vi "Example - Class.vi"() -> ()   [LabVIEW 2020]
uses:
  1d4a776c-2696-3fe4-d0bb-77cddb30cb3f.vi
  3faee846-98d4-3fe1-9c43-23fda36bd13f.vi
  b5272922-ba09-3fe1-f861-5bbbaacdd13f.vi
  EquipmentVariant/Type Enum.ctl
  EquipmentVariant/EquipmentVariant.lvclass
  fdb528fa-7372-3fe0-10ac-5ff425bcdf3f.vi
  49be02a8-6884-3fd8-d48e-5d860b02e23f.vi
  cd560766-33b7-3fed-e07d-7da03414de3f.vi
  d5be5900-83d0-3fd0-7918-a6c719c6ef3f.vi
  70d5f8a8-1432-3fec-90d8-8f9e559dd13f.vi
  6e1ed180-022c-3fcd-f5ed-a54cfad1e83f.vi
  092b700a-44bb-3fe9-485c-b2951c1cd43f.vi
  43438abc-0b96-3fe5-e002-a3a3c6ecc43f.vi
  682f44c6-7f56-3fe3-7cfd-dfadc80bee3f.vi
  2733e0e4-24d6-3fee-700d-63818caedb3f.vi
  915d7a80-1a4e-3fce-50ff-63604885b63f.vi
  Robot/Robot.lvclass
  Pump/Pump.lvclass
  45b58a9c-ccc2-3fe8-f4b2-f6788901e33f.vi
  36c48e48-6b2d-3fef-c04d-7500d28fc73f.vi
  507d9734-094a-3fee-fad7-d41d2ba6e43f.vi
  home/jki/Projects/enumerated-variant-labview-idea/source/EnumeratedVariant/EnumeratedVariant.lvclass
  home/jki/Projects/enumerated-variant-labview-idea/source/EquipmentVariant/EquipmentVariant.lvclass
  75226f00-6cff-3fc0-1085-64b70facdd3f.vi
  1b391bf8-c4d0-3fd5-10eb-bf28fd58bc3f.vi
  dfc18360-e89b-3fe8-f7d0-384086f7e73f.vi
  a19e52fe-f2f8-3fee-80fa-777f1c989c3f.vi
  b0de32f8-392d-3fea-f061-38c88206d93f.vi
  47083128-469b-3fd6-4083-c0c0298ca53f.vi
  f64f6dae-26cd-3fe7-164d-c343c130e33f.vi
  d52d8690-3443-3fb2-48a2-82c20901ea3f.vi
  9c66e4d8-756c-3fe3-f899-0197e0a0e13f.vi
  fbe86e10-61e9-3fd4-3453-d6eec0f7ec3f.vi
  bcedb830-bb68-3fd0-605d-ec66737db43f.vi
  9f07b280-4224-3fc7-a086-75c6439fc93f.vi
  efe137e0-dc7b-3fc0-d86a-56f12716df3f.vi
  5fb9f880-a967-3fa0-c07e-0f50a7d0c93f.vi
  65dfe200-eb14-3fe5-806e-08bf00ddc13f.vi
panel:
  in  "error in":errorcluster
  out "error out":errorcluster
  out "Pump 3":refnum<class "Pump.lvclass">
  out "Robot 4":refnum<class "Robot.lvclass">
  out "Equipment Array":refnum<class "EquipmentVariant.lvclass">[](array[class])
  out "Pump 2":refnum<class "Pump.lvclass">
  out "Robot 3":refnum<class "Robot.lvclass">
  out "Pump":refnum<class "Pump.lvclass">
  out "Robot 2":refnum<class "Robot.lvclass">
  out "Pump":refnum<class "Pump.lvclass">
  out "Robot":refnum<class "Robot.lvclass">
  out "Pump":refnum<class "Pump.lvclass">
  out "Robot":refnum<class "Robot.lvclass">
  out "specific type":refnum<visa-resource-name>="abc"
  out "specific type":refnum<class "Pump.lvclass">
  out "specific type":refnum<class "Robot.lvclass">
  out "Pump":refnum<class "Pump.lvclass">
  out "Robot":refnum<class "Robot.lvclass">
  out "Pump":refnum<class "Pump.lvclass">
  out "Robot":refnum<class "Robot.lvclass">
  out "Equivalent?":bool
  out "Equivalent?":bool
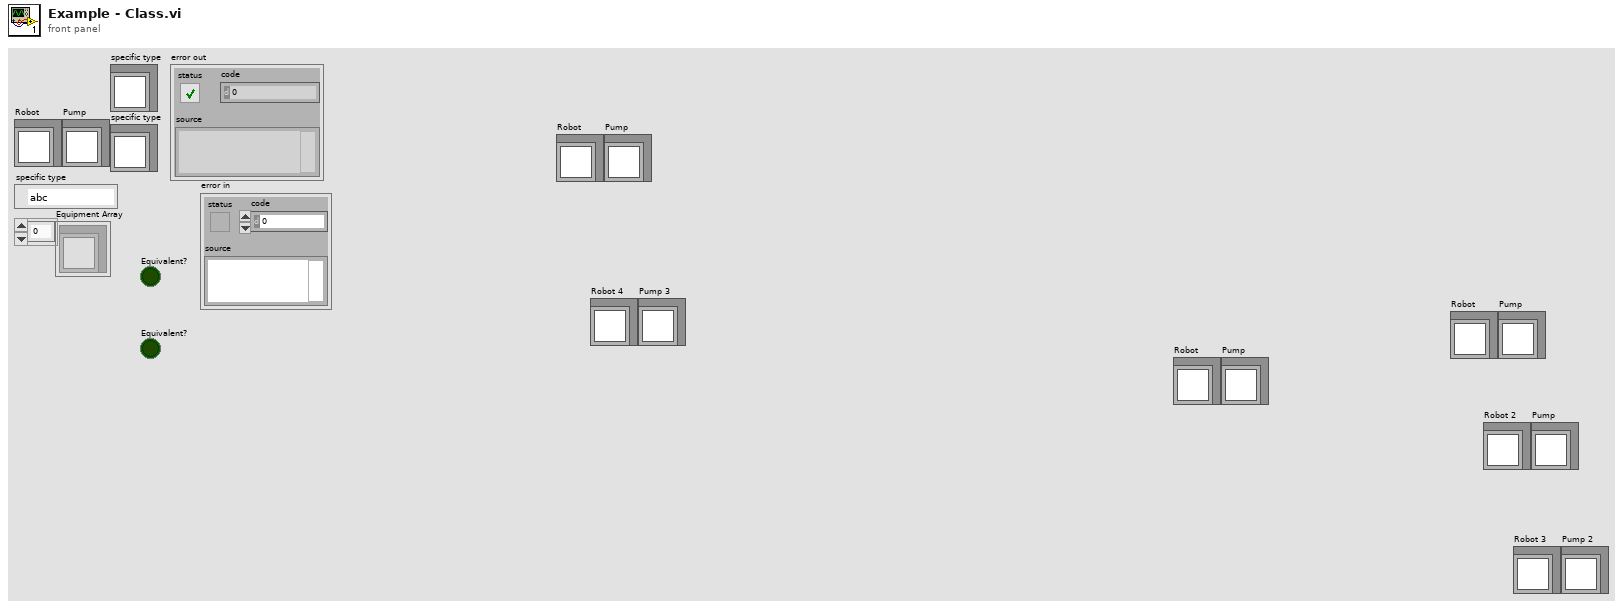
[diagram p1: front panel]
types:
  T1 = typedef "EquipmentVariant.lvclass/Type Enum.ctl" = enum16{"Robot", "Pump", "Instrument"}
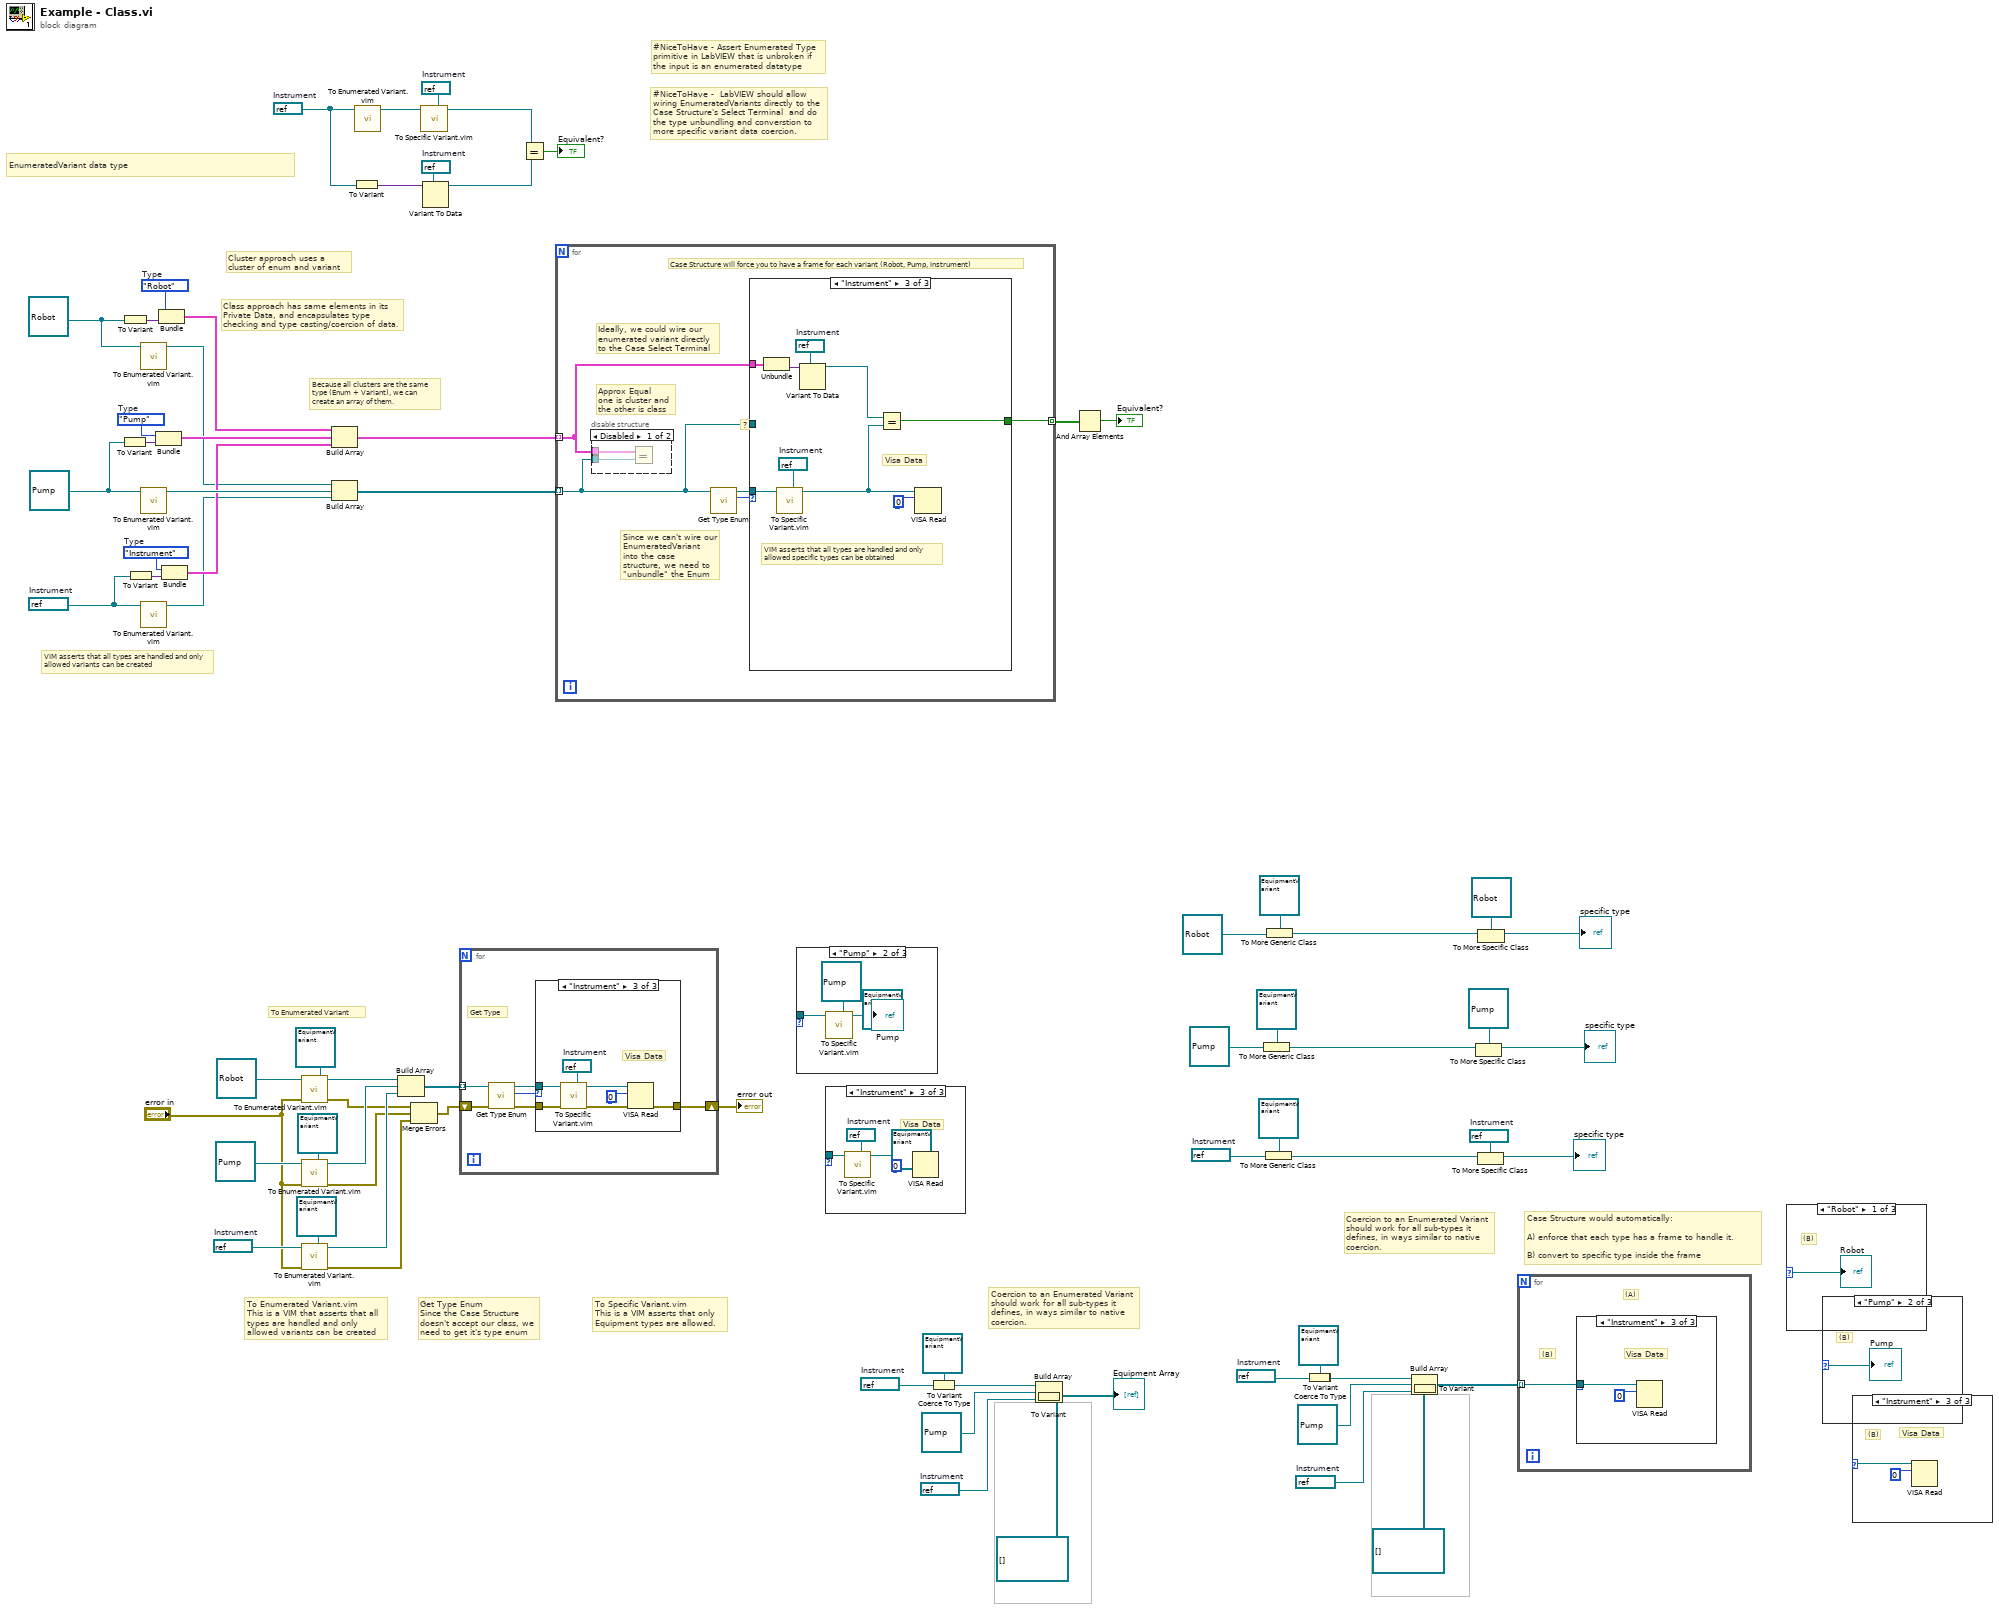
[diagram p0: block diagram]
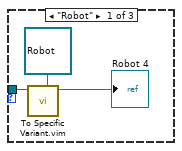
[diagram p2: hidden frame]
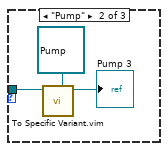
[diagram p3: hidden frame]
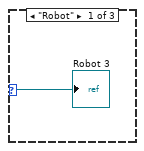
[diagram p4: hidden frame]
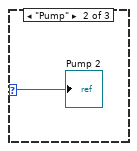
[diagram p5: hidden frame]
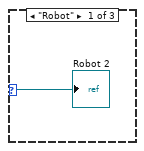
[diagram p6: hidden frame]
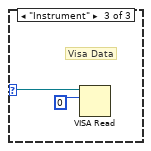
[diagram p7: hidden frame]
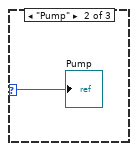
[diagram p8: hidden frame]
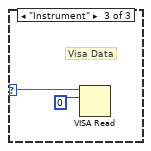
[diagram p9: hidden frame]
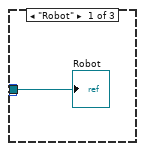
[diagram p10: hidden frame]
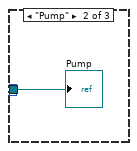
[diagram p11: hidden frame]
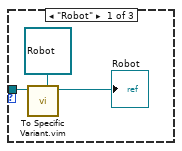
[diagram p12: hidden frame]
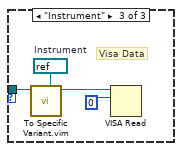
[diagram p13: hidden frame]
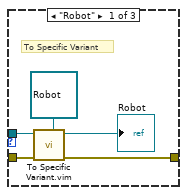
[diagram p14: hidden frame]
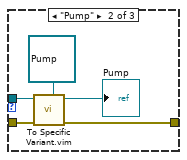
[diagram p15: hidden frame]
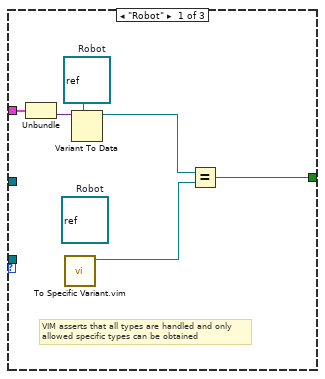
[diagram p17: hidden frame]
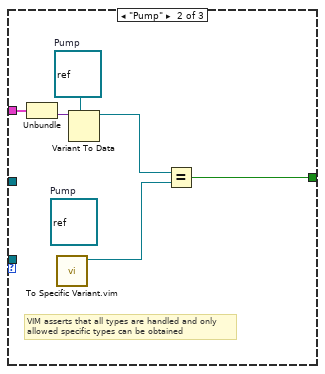
[diagram p18: hidden frame]
diagram:
  w14 = refnum<visa-resource-name> "abc"  # Instrument
  w10 = refnum<visa-resource-name> "abc"  # Instrument
  w16 = refnum<visa-resource-name> "abc"  # Instrument
  w20 = refnum<visa-resource-name> "abc"  # Instrument
  w23 = refnum<visa-resource-name> "abc"  # Instrument
  w24 = refnum<visa-resource-name> "abc"  # Instrument
  w8 = refnum<class "Robot.lvclass"> refnum ("Robot.lvclass")
  w40 = refnum<class "Pump.lvclass"> refnum ("Pump.lvclass")
  w43 = refnum<visa-resource-name> "abc"  # Instrument
  w54 = refnum<visa-resource-name> refnum  # Instrument
  w48 = refnum<visa-resource-name> refnum  # Instrument
  w56 = refnum<visa-resource-name> refnum  # Instrument
  w68 = Type_Enum."Instrument"  # Type
  w69 = Type_Enum."Pump"  # Type
  w70 = Type_Enum."Robot"  # Type
  w49 = refnum<visa-resource-name> "abc"  # Instrument
  # "To Enumerated Variant"
  # "Coercion to an Enumerated Variant should work for all sub-types it defines, in ways similar to native coercion."
  # "Case Structure would automatically:\n\nA) enforce that each type has a frame to handle it.\n\nB) convert to specific type inside the frame"
  # "Coercion to an Enumerated Variant should work for all sub-types it defines, in ways similar to native coercion."
  # "Get Type Enum\nSince the Case Structure doesn't accept our class, we need to get it's type enum"
  # "To Specific Variant.vim\nThis is a VIM asserts that only Equipment types are allowed."
  # "To Enumerated Variant.vim\nThis is a VIM that asserts that all types are handled and only allowed variants can be created"
  # "#NiceToHave - Assert Enumerated Type primitive in LabVIEW that is unbroken if the input is an enumerated datatype"
  # "VIM asserts that all types are handled and only allowed variants can be created"
  # "Class approach has same elements in its Private Data, and encapsulates type checking and type casting/coercion of data."
  # "Cluster approach uses a cluster of enum and variant"
  # "#NiceToHave -  LabVIEW should allow wiring EnumeratedVariants directly to the Case Structure's Select Terminal  and do the type unbundling and converstion to more specific variant data coercion."
  # "Because all clusters are the same type (Enum + Variant), we can create an array of them."
  # "EnumeratedVariant data type"
  n1 = To Variant(anything=w40) -> (Variant=w60:variant)
  n2 = To Variant(anything=w8) -> (Variant=w71:variant)
  n3 = To Variant(anything=w49) -> (Variant=w59:variant)
  n4 = call "To Enumerated Variant.vim"("Type"=w8) -> ("EquipmentVariant"=w58:refnum<class "EquipmentVariant.lvclass">)  [unwired: 9 in, 1 out]
  n5 = call "To Enumerated Variant.vim"("Type"=w40) -> ("EquipmentVariant"=w67:refnum<class "EquipmentVariant.lvclass">)  [unwired: 9 in, 1 out]
  n6 = call "To Enumerated Variant.vim"("Type"=w49) -> ("EquipmentVariant"=w50:refnum<class "EquipmentVariant.lvclass">)  [unwired: 9 in, 1 out]
  n7 = Bundle("Type"=w69, "Variant"=w60) -> (w66:cluster{"Type":T1, "Variant":variant})  [unwired: 1 in]
  n8 = Bundle("Type"=w70, "Variant"=w71) -> (w63:cluster{"Type":T1, "Variant":variant})  [unwired: 1 in]
  n9 = Bundle("Type"=w68, "Variant"=w59) -> (w65:cluster{"Type":T1, "Variant":variant})  [unwired: 1 in]
  n10 = call "To Enumerated Variant.vim"("Enumerated Type"=refnum<class "EquipmentVariant.lvclass"> refnum ("EquipmentVariant"), "error in"="error in", "Type"=refnum<class "Robot.lvclass"> refnum ("Robot.lvclass")) -> ("error out"=w6:errorcluster, "EquipmentVariant"=w45:refnum<class "EquipmentVariant.lvclass">)  [unwired: 7 in]
  n11 = call "To Enumerated Variant.vim"("Enumerated Type"=refnum<class "EquipmentVariant.lvclass"> refnum ("EquipmentVariant"), "error in"="error in", "Type"=refnum<class "Pump.lvclass"> refnum ("Pump.lvclass")) -> ("error out"=w4:errorcluster, "EquipmentVariant"=w46:refnum<class "EquipmentVariant.lvclass">)  [unwired: 7 in]
  n12 = call "To Enumerated Variant.vim"("Enumerated Type"=refnum<class "EquipmentVariant.lvclass"> refnum ("EquipmentVariant"), "error in"="error in", "Type"=w43) -> ("error out"=w3:errorcluster, "EquipmentVariant"=w44:refnum<class "EquipmentVariant.lvclass">)  [unwired: 7 in]
  n13 = Build Array(w63, w66, w65) -> (w64:cluster{"Type":T1, "Variant":variant}[])
  n14 = Build Array(w58, w67, w50) -> (w72:refnum<class "EquipmentVariant.lvclass">[])
  n15 = To Variant(anything=w56) -> (Variant=w55:variant)
  n16 = call "To Enumerated Variant.vim"("Type"=w56) -> ("EquipmentVariant"=w57:refnum<class "EquipmentVariant.lvclass">)  [unwired: 9 in, 1 out]
  n17 = Build Array(w45, w46, w44) -> (w47:refnum<class "EquipmentVariant.lvclass">[])
  n18 = Merge Errors(w6, w4, w3) -> (w5:errorcluster)
  n19 = call "To Specific Variant.vim"("Type"=w48, "EquipmentVariant.lvclass"=w57) -> ("Specific Variant"=w53:refnum<visa-resource-name>)  [unwired: 8 in, 1 out]
  n20 = Variant To Data(type=w54, Variant=w55) -> (data=w52:refnum<visa-resource-name>)  [unwired: 1 in, 1 out]
  n21 = for {
    tunnel: w47 -> [w77] mode=indexing
    shift-right: [w73] -> w2
    shift-left: w5 -> [w75]
    # "Get Type"
    n22 = call "Get Type Enum.vi"("error in (no error)"=w75, "EquipmentVariant in"=w77) -> ("error out"=w74:errorcluster, "Type"=w76:T1, "EquipmentVariant out"=w78:refnum<class "EquipmentVariant.lvclass">)  [unwired: 7 in]
    n23 = case shown="\"Instrument\"" w76 {
      tunnel: w78 -> [w83 w88 w94]
      tunnel: w74 -> [w80 w85 w90]
      tunnel: [w79 w84 w89] -> w73
      frame "Robot" {
        # "To Specific Variant"
        n24 = call "To Specific Variant.vim"("Type"=refnum<class "Robot.lvclass"> refnum ("Robot.lvclass"), "error in"=w80, "EquipmentVariant.lvclass"=w83) -> ("error out"=w79:errorcluster, "Specific Variant"=→"Robot":refnum<class "Robot.lvclass">)  [unwired: 7 in]
      }
      frame "Pump" {
        n25 = call "To Specific Variant.vim"("Type"=refnum<class "Pump.lvclass"> refnum ("Pump.lvclass"), "error in"=w85, "EquipmentVariant.lvclass"=w88) -> ("error out"=w84:errorcluster, "Specific Variant"=→"Pump":refnum<class "Pump.lvclass">)  [unwired: 7 in]
      }
      frame "Instrument" {
        w92 = refnum<visa-resource-name> refnum  # Instrument
        # "Visa Data"
        n26 = call "To Specific Variant.vim"("Type"=w92, "error in"=w90, "EquipmentVariant.lvclass"=w94) -> ("error out"=w91:errorcluster, "Specific Variant"=w93:refnum<visa-resource-name>)  [unwired: 7 in]
        n27 = VISA Read(VISA resource name=w93, byte count=u32 0, error in (no error)=w91) -> (error out=w89:errorcluster)  [unwired: 3 out]
      }
    }
  }
  "error out" <- w2
  n28 = Equal?(x=w53, y=w52) -> (x = y?=→"Equivalent?":bool)
  n29 = for {
    tunnel: w72 -> [w96] mode=indexing
    tunnel: w64 -> [w99] mode=indexing
    tunnel: [w100] -> w62 mode=indexing
    # "?"
    # "Ideally, we could wire our enumerated variant directly to the Case Select Terminal"
    # "Approx Equal\none is cluster and the other is class"
    # "Since we can't wire our EnumeratedVariant into the case structure, we need to \"unbundle\" the Enum"
    # "Case Structure will force you to have a frame for each variant (Robot, Pump, Instrument)"
    n30 = disable-structure shown="Disabled" {
      disable-tunnel: w96 -> [w102 _]
      disable-tunnel: w99 -> [w101 _]
      frame Disabled {
        n31 = Equal?(x=w101, y=w102) -> ()  [unwired: 1 out]
      }
      frame Enabled {
      }
    }
    n32 = call "Get Type Enum.vi"("EquipmentVariant in"=w96) -> ("Type"=w98:T1, "EquipmentVariant out"=w97:refnum<class "EquipmentVariant.lvclass">)  [unwired: 8 in, 1 out]
    n33 = case shown="\"Instrument\"" w98 {
      tunnel: w97 -> [_ _ w117]
      tunnel: [w105 w112 w120] -> w100
      tunnel: w99 -> [w104 w110 w119]
      tunnel: w96 -> [_ _ _]
      frame "Robot" {
        w108 = refnum<class> refnum  # Robot
        (unwired) refnum<class> refnum  # Robot
        # "VIM asserts that all types are handled and only allowed specific types can be obtained"
        n34 = Unbundle(w104) -> ("Variant"=w103:variant)  [unwired: 1 out]
        n35 = call "To Specific Variant.vim"() -> ("Specific Variant"=w106:refnum<class "Robot.lvclass">)  [unwired: 10 in, 1 out]
        n36 = Variant To Data(type=w108, Variant=w103) -> (data=w107:refnum<class>)  [unwired: 1 in, 1 out]
        n37 = Equal?(x=w107, y=w106) -> (x = y?=w105:bool)
      }
      frame "Pump" {
        w111 = refnum<class> refnum  # Pump
        (unwired) refnum<class> refnum  # Pump
        # "VIM asserts that all types are handled and only allowed specific types can be obtained"
        n38 = Unbundle(w110) -> ("Variant"=w109:variant)  [unwired: 1 out]
        n39 = call "To Specific Variant.vim"() -> ("Specific Variant"=w113:refnum<class "Robot.lvclass">)  [unwired: 10 in, 1 out]
        n40 = Variant To Data(type=w111, Variant=w109) -> (data=w114:refnum<class>)  [unwired: 1 in, 1 out]
        n41 = Equal?(x=w114, y=w113) -> (x = y?=w112:bool)
      }
      frame "Instrument" {
        w122 = refnum<visa-resource-name> refnum  # Instrument
        w115 = refnum<visa-resource-name> refnum  # Instrument
        # "VIM asserts that all types are handled and only allowed specific types can be obtained"
        # "Visa Data"
        n42 = Unbundle(w119) -> ("Variant"=w118:variant)  [unwired: 1 out]
        n43 = call "To Specific Variant.vim"("Type"=w115, "EquipmentVariant.lvclass"=w117) -> ("Specific Variant"=w116:refnum<visa-resource-name>)  [unwired: 8 in, 1 out]
        n44 = Variant To Data(type=w122, Variant=w118) -> (data=w121:refnum<visa-resource-name>)  [unwired: 1 in, 1 out]
        n45 = Equal?(x=w121, y=w116) -> (x = y?=w120:bool)
        n46 = VISA Read(VISA resource name=w116, byte count=u32 0) -> ()  [unwired: 1 in, 4 out]
      }
    }
  }
  n47 = case shown="\"Pump\"" {
    selector: _ -> [_ _ _]
    tunnel: refnum<class "EquipmentVariant.lvclass"> refnum ("EquipmentVariant.lvclass") -> [w126 w129 w132]
    frame "Robot" {
      n48 = call "To Specific Variant.vim"("Type"=refnum<class "Robot.lvclass"> refnum ("Robot.lvclass"), "EquipmentVariant.lvclass"=w126) -> ("Specific Variant"=→"Robot":refnum<class "Robot.lvclass">)  [unwired: 8 in, 1 out]
    }
    frame "Pump" {
      n49 = call "To Specific Variant.vim"("Type"=refnum<class "Pump.lvclass"> refnum ("Pump.lvclass"), "EquipmentVariant.lvclass"=w129) -> ("Specific Variant"=→"Pump":refnum<class "Pump.lvclass">)  [unwired: 8 in, 1 out]
    }
    frame "Instrument" {
      w130 = refnum<visa-resource-name> refnum  # Instrument
      # "Visa Data"
      n50 = call "To Specific Variant.vim"("Type"=w130, "EquipmentVariant.lvclass"=w132) -> ("Specific Variant"=w131:refnum<visa-resource-name>)  [unwired: 8 in, 1 out]
      n51 = VISA Read(VISA resource name=w131, byte count=u32 0) -> ()  [unwired: 1 in, 4 out]
    }
  }
  n52 = case shown="\"Instrument\"" {
    selector: _ -> [_ _ _]
    tunnel: refnum<class "EquipmentVariant.lvclass"> refnum ("EquipmentVariant.lvclass") -> [w136 w139 w142]
    frame "Robot" {
      n53 = call "To Specific Variant.vim"("Type"=refnum<class "Robot.lvclass"> refnum ("Robot.lvclass"), "EquipmentVariant.lvclass"=w136) -> ("Specific Variant"=→"Robot 4":refnum<class "Robot.lvclass">)  [unwired: 8 in, 1 out]
    }
    frame "Pump" {
      n54 = call "To Specific Variant.vim"("Type"=refnum<class "Pump.lvclass"> refnum ("Pump.lvclass"), "EquipmentVariant.lvclass"=w139) -> ("Specific Variant"=→"Pump 3":refnum<class "Pump.lvclass">)  [unwired: 8 in, 1 out]
    }
    frame "Instrument" {
      w140 = refnum<visa-resource-name> refnum  # Instrument
      # "Visa Data"
      n55 = call "To Specific Variant.vim"("Type"=w140, "EquipmentVariant.lvclass"=w142) -> ("Specific Variant"=w141:refnum<visa-resource-name>)  [unwired: 8 in, 1 out]
      n56 = VISA Read(VISA resource name=w141, byte count=u32 0) -> ()  [unwired: 1 in, 4 out]
    }
  }
  n57 = Coerce To Type(1:refnum<class "EquipmentVariant.lvclass"> refnum ("EquipmentVariant")) -> (2:w12:refnum<class "EquipmentVariant.lvclass">)  [unwired: 1 in]
  n58 = To Variant(anything=w10) -> ()  [unwired: 1 out]
  n59 = Build Array(w12, refnum<class "Pump.lvclass"> refnum ("Pump.lvclass")) -> ()  [unwired: 1 in, 1 out]
  n60 = To Variant(anything=w14) -> ()  [unwired: 1 out]
  n61 = And Array Elements(Boolean array=w62) -> (logical AND=→"Equivalent?":bool)
  n62 = To More Generic Class(target class=refnum<class "EquipmentVariant.lvclass"> refnum ("EquipmentVariant"), reference=refnum<class "Pump.lvclass"> refnum ("Pump.lvclass")) -> (generic class reference=w30:refnum<class "EquipmentVariant.lvclass">)
  n63 = To More Generic Class(target class=refnum<class "EquipmentVariant.lvclass"> refnum ("EquipmentVariant"), reference=w24) -> (generic class reference=w25:refnum<class "EquipmentVariant.lvclass">)
  n64 = To More Generic Class(target class=refnum<class "EquipmentVariant.lvclass"> refnum ("EquipmentVariant"), reference=refnum<class "Robot.lvclass"> refnum ("Robot.lvclass")) -> (generic class reference=w32:refnum<class "EquipmentVariant.lvclass">)
  n65 = Coerce To Type(1:refnum<class "EquipmentVariant.lvclass"> refnum ("EquipmentVariant")) -> (2:w18:refnum<class "EquipmentVariant.lvclass">)  [unwired: 1 in]
  n66 = To Variant(anything=w20) -> ()  [unwired: 1 out]
  n67 = Build Array(w18, refnum<class "Pump.lvclass"> refnum ("Pump.lvclass")) -> ()  [unwired: 1 in, 1 out]
  n68 = To Variant(anything=w16) -> ()  [unwired: 1 out]
  n69 = To More Specific Class(target class=refnum<class "Pump.lvclass"> refnum ("Pump.lvclass"), reference=w30) -> (specific class reference=→"specific type":refnum<class "Pump.lvclass">)  [unwired: 1 in, 1 out]
  n70 = To More Specific Class(target class=w23, reference=w25) -> (specific class reference=→"specific type":refnum<class "EquipmentVariant.lvclass">)  [unwired: 1 in, 1 out]
  n71 = To More Specific Class(target class=refnum<class "Robot.lvclass"> refnum ("Robot.lvclass"), reference=w32) -> (specific class reference=→"specific type":refnum<class "Robot.lvclass">)  [unwired: 1 in, 1 out]
  n72 = for {
    tunnel: refnum<class "EquipmentVariant.lvclass">[] [] ("appended array") -> [w144] mode=indexing
    # "(A)"
    # "(B)"
    n73 = case shown="\"Instrument\"" {
      selector: _ -> [_ _ _]
      tunnel: w144 -> [w147 w150 w153]
      frame "Robot" {
        n74 = call "To Specific Variant.vim"("Type"=refnum<class "Robot.lvclass"> refnum ("Robot.lvclass"), "EquipmentVariant.lvclass"=w147) -> ("Specific Variant"=→"Robot":refnum<class "Robot.lvclass">)  [unwired: 8 in, 1 out]
      }
      frame "Pump" {
        n75 = call "To Specific Variant.vim"("Type"=refnum<class "Pump.lvclass"> refnum ("Pump.lvclass"), "EquipmentVariant.lvclass"=w150) -> ("Specific Variant"=→"Pump":refnum<class "Pump.lvclass">)  [unwired: 8 in, 1 out]
      }
      frame "Instrument" {
        w151 = refnum<visa-resource-name> refnum  # Instrument
        # "Visa Data"
        n76 = call "To Specific Variant.vim"("Type"=w151, "EquipmentVariant.lvclass"=w153) -> ("Specific Variant"=w152:refnum<visa-resource-name>)  [unwired: 8 in, 1 out]
        n77 = VISA Read(VISA resource name=w152, byte count=u32 0) -> ()  [unwired: 1 in, 4 out]
      }
    }
  }
  n78 = case shown="\"Robot\"" {
    selector: _ -> [_ _ _]
    frame "Robot" {
      # "(B)"
      n79 = call "To Specific Variant.vim"("Type"=refnum<class "Robot.lvclass"> refnum ("Robot.lvclass")) -> ("Specific Variant"=→"Robot":refnum<class "Robot.lvclass">)  [unwired: 9 in, 1 out]
    }
    frame "Pump" {
      n80 = call "To Specific Variant.vim"("Type"=refnum<class "Pump.lvclass"> refnum ("Pump.lvclass")) -> ("Specific Variant"=→"Pump":refnum<class "Pump.lvclass">)  [unwired: 9 in, 1 out]
    }
    frame "Instrument" {
      w159 = refnum<visa-resource-name> refnum  # Instrument
      # "Visa Data"
      n81 = call "To Specific Variant.vim"("Type"=w159) -> ("Specific Variant"=w160:refnum<visa-resource-name>)  [unwired: 9 in, 1 out]
      n82 = VISA Read(VISA resource name=w160, byte count=u32 0) -> ()  [unwired: 1 in, 4 out]
    }
  }
  n83 = case shown="\"Pump\"" {
    selector: _ -> [_ _ _]
    frame "Robot" {
      n84 = call "To Specific Variant.vim"("Type"=refnum<class "Robot.lvclass"> refnum ("Robot.lvclass")) -> ("Specific Variant"=→"Robot 2":refnum<class "Robot.lvclass">)  [unwired: 9 in, 1 out]
    }
    frame "Pump" {
      # "(B)"
      n85 = call "To Specific Variant.vim"("Type"=refnum<class "Pump.lvclass"> refnum ("Pump.lvclass")) -> ("Specific Variant"=→"Pump":refnum<class "Pump.lvclass">)  [unwired: 9 in, 1 out]
    }
    frame "Instrument" {
      w166 = refnum<visa-resource-name> refnum  # Instrument
      # "Visa Data"
      n86 = call "To Specific Variant.vim"("Type"=w166) -> ("Specific Variant"=w167:refnum<visa-resource-name>)  [unwired: 9 in, 1 out]
      n87 = VISA Read(VISA resource name=w167, byte count=u32 0) -> ()  [unwired: 1 in, 4 out]
    }
  }
  n88 = case shown="\"Instrument\"" {
    selector: _ -> [_ _ _]
    frame "Robot" {
      n89 = call "To Specific Variant.vim"("Type"=refnum<class "Robot.lvclass"> refnum ("Robot.lvclass")) -> ("Specific Variant"=→"Robot 3":refnum<class "Robot.lvclass">)  [unwired: 9 in, 1 out]
    }
    frame "Pump" {
      n90 = call "To Specific Variant.vim"("Type"=refnum<class "Pump.lvclass"> refnum ("Pump.lvclass")) -> ("Specific Variant"=→"Pump 2":refnum<class "Pump.lvclass">)  [unwired: 9 in, 1 out]
    }
    frame "Instrument" {
      w173 = refnum<visa-resource-name> refnum  # Instrument
      # "(B)"
      # "Visa Data"
      n91 = call "To Specific Variant.vim"("Type"=w173) -> ("Specific Variant"=w174:refnum<visa-resource-name>)  [unwired: 9 in, 1 out]
      n92 = VISA Read(VISA resource name=w174, byte count=u32 0) -> ()  [unwired: 1 in, 4 out]
    }
  }
  "Equipment Array" <- refnum<class "EquipmentVariant.lvclass">[] [] ("appended array")
